vi "barcode tester.vi"() -> ()   [LabVIEW 2025]
uses:
  <vilib>/Instr/_visa.llb/VISA Configure Serial Port (Instr).vi
panel:
  out "unsigned byte array":u8[](array[numeric])
  out "read buffer":string
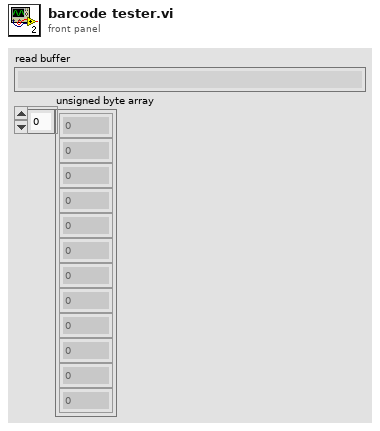
[diagram p1: front panel]
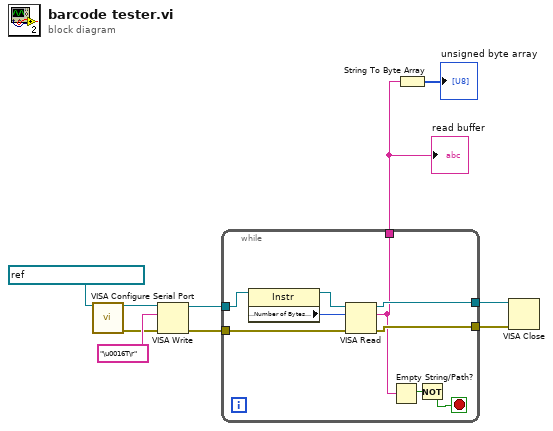
[diagram p0: block diagram]
diagram:
  n1 = call-poly "VISA Configure Serial Port"("VISA resource name"=refnum<visa-resource-name> "BARCODE_RECEIVER") -> ("VISA resource name out"=w7:refnum<visa-resource-name>, "error out"=w8:errorcluster)  [unwired: 13 in]
  n2 = VISA Write(VISA resource name=w7, write buffer="\u0016T\r", error in (no error)=w8) -> (VISA resource name out=w5:refnum<visa-resource-name>, error out=w6:errorcluster)  [unwired: 1 out]
  n3 = while {
    tunnel: w6 -> [w15]
    tunnel: w5 -> [w14]
    tunnel: [w13] -> w4
    tunnel: [w12] -> w3
    tunnel: [w11] -> w2
    stop <- w16 stop-if-true
    n4 = property class="Instr"(reference=w14) -> (reference out=w19:refnum<visa-resource-name>, "Serial Settings:Number of Bytes at Serial Port"=w18:u32)  [unwired: 1 in, 1 out]
    n5 = VISA Read(VISA resource name=w19, byte count=w18, error in (no error)=w15) -> (VISA resource name out=w12:refnum<visa-resource-name>, read buffer=w11:string, error out=w13:errorcluster)  [unwired: 1 out]
    n6 = Empty String/Path?(string/path=w11) -> (empty?=w17:bool)
    n7 = Not(x=w17) -> (.not. x?=w16:bool)
  }
  "read buffer" <- w2
  n8 = String To Byte Array(string=w2) -> (unsigned byte array=→"unsigned byte array":u8[])
  n9 = VISA Close(VISA resource name=w3, error in (no error)=w4) -> ()  [unwired: 1 out]
